vi "TXT Global.vi"() -> ()   [LabVIEW 2017, in "TXT.lvlib" / "TXT.lvclass"]
uses:
  TXT.lvclass
panel:
  in  "End File Section":string="End:::"
  in  "Start File Section":string="Start:"
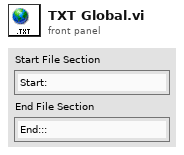
[diagram p1: front panel]
diagram:
